vi "Make_Tree_Item.vi"(8 "error in (no error)":errorcluster, 11 "IB_RestfulWS in":refnum<class "IB_RestfulWS.lvclass">) -> (0 "error out":errorcluster, 3 "TreeSrcItem":refnum<class "IB_Tree_Item_Source.lvclass">)   [LabVIEW 2020, in "IB_RestfulWS.lvclass"]
uses:
  <vilib>/AppBuilder/IB_Classes/Source/Container/Build/RestfulWS/IB_RestfulWS.lvclass
  <vilib>/AppBuilder/IB_Classes/Source/Container/Build/RestfulWS/IB_RestfulWS.lvclass/IB_RestfulWS.ctl
  <vilib>/AppBuilder/IB_Classes/Tree_Item_Source_RestfulWS/IB_Tree_Item_Source_RestfulWS.lvclass
  e:/builds/penguin/labview/branches/2020/dev/dist/vi.lib/AppBuilder/IB_Classes/Source/Container/Build/IB_Source_Build.lvclass
  e:/builds/penguin/labview/branches/2020/dev/dist/vi.lib/AppBuilder/IB_Classes/Source/Container/IB_Source_Container.lvclass
  e:/builds/penguin/labview/branches/2020/dev/dist/vi.lib/AppBuilder/IB_Classes/Source/IB_Source.lvclass
  e:/builds/penguin/labview/branches/2020/dev/dist/vi.lib/AppBuilder/IB_Classes/Source/Container/Build/RestfulWS/IB_RestfulWS.lvclass
  e:/builds/penguin/labview/branches/2020/dev/dist/vi.lib/AppBuilder/IB_Classes/Tree_Item_Source_Build/IB_Tree_Item_Source_Build.lvclass
  e:/builds/penguin/labview/branches/2020/dev/dist/vi.lib/AppBuilder/IB_Classes/Tree_Item_Source_Container/IB_Tree_Item_Source_Container.lvclass
  e:/builds/penguin/labview/branches/2020/dev/dist/vi.lib/AppBuilder/IB_Classes/Tree_Item_Source/IB_Tree_Item_Source.lvclass
  e:/builds/penguin/labview/branches/2020/dev/dist/vi.lib/AppBuilder/IB_Classes/Tree_Item/IB_Tree_Item.lvclass
  e:/builds/penguin/labview/branches/2020/dev/dist/vi.lib/AppBuilder/IB_Classes/Tree_Item_Source_RestfulWS/IB_Tree_Item_Source_RestfulWS.lvclass
  <vilib>/AppBuilder/IB_Classes/Tree_Item_Source/IB_Tree_Item_Source.lvclass
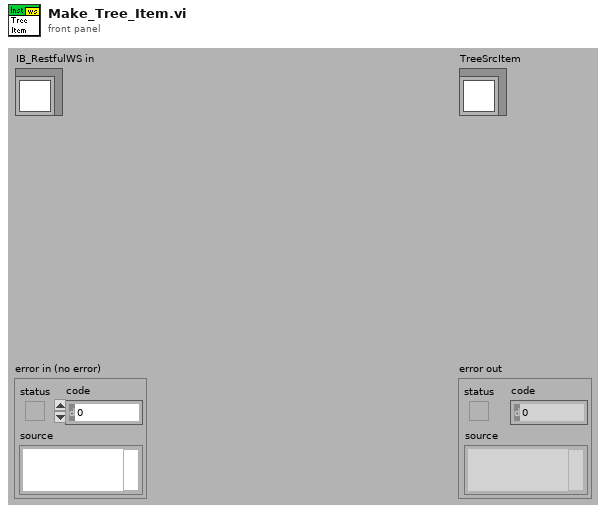
[diagram p1: front panel]
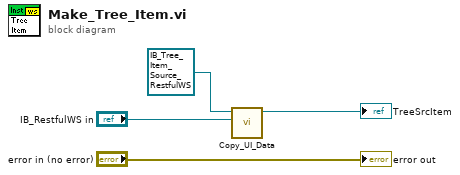
[diagram p0: block diagram]
diagram:
  n1 = call-dynamic "Copy_UI_Data.vi"("IB_Source in"="IB_RestfulWS in", "IB_TreeContainerItem.lvclass"=refnum<class "IB_Tree_Item_Source_RestfulWS.lvclass"> refnum ("IB_Tree_Item_Source_RestfulWS.lvclass")) -> ("IB_TreeContainerItem out"=→"TreeSrcItem":refnum<class "IB_Tree_Item_Source_RestfulWS.lvclass">)  [unwired: 1 in, 8 out]
  "error out" <- "error in (no error)"
